vi "심플 엣지 카운트.vi"() -> ()   [LabVIEW 2018]
uses:
  <vilib>/DAQmx/read.llb/DAQmx Read (Counter DBL 1Chan 1Samp).vi
  <vilib>/DAQmx/create/channels.llb/DAQmx Create Channel (CI-Count Edges).vi
  <vilib>/DAQmx/miscellaneous.llb/DAQmx Fill In Error Info.vi
panel:
  in  "정지 버튼":bool
  out "data 2":dbl caption="데이터" format="%0.2f"
  in  "edge":i32(ring)=10280 caption="에지" items=["상승"=10280, "하강"=10171]
  in  "count direction":i32(ring)=10128 caption="카운트 방향" items=["카운트 업"=10128, "카운트 다운"=10124, "외부 컨트롤"=10326]
  in  "initial count":u32 caption="초기 카운트"
  in  "counter":tag caption="카운터"
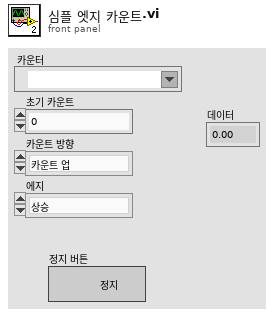
[diagram p1: front panel]
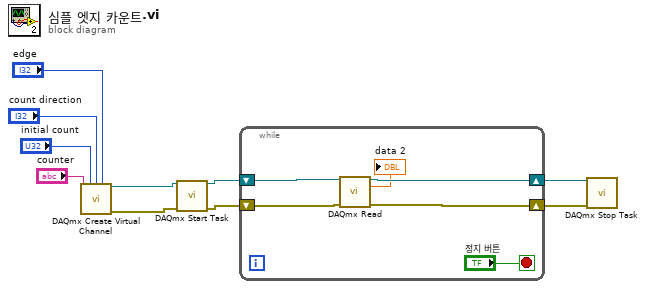
[diagram p0: block diagram]
diagram:
  n1 = call-poly <vilib>:"DAQmx Create Virtual Channel.vi"("initial count"="initial count", "count direction"="count direction", "edge"="edge", "counter"="counter") -> ("task out"=w10:refnum<k21>, "error out"=w9:errorcluster)  [unwired: 10 in]
  n2 = call <vilib>:"DAQmx Start Task.vi"("task/channels in"=w10, "error in"=w9) -> ("task out"=w7:refnum<k21>, "error out"=w8:errorcluster)  [unwired: 12 in]
  n3 = while {
    shift-right: [w13] -> w5
    shift-left: w8 -> [w16]
    shift-right: [w14] -> w6
    shift-left: w7 -> [w15]
    stop <- "정지 버튼" stop-if-true
    n4 = call-poly <vilib>:"DAQmx Read.vi"("task/channels in"=w15, "error in"=w16) -> ("task out"=w14:refnum<k21>, "data"=→"data 2":dbl, "error out"=w13:errorcluster)  [unwired: 11 in]
  }
  n5 = call <vilib>:"DAQmx Stop Task.vi"("task/channels in"=w6, "error in"=w5) -> ()  [unwired: 12 in, 2 out]
